vi "Calculate Time and Date.vi"() -> (1 "Date":dbl, 3 "Time":dbl)   [LabVIEW 2018]
doc: "OSDS Calculate Time and Date.vi\n\n This VI calculates the time and date as double based on the time stamp.\n\nOCC Streaming Data System Version 1.0\nJune, 2007 Original Code Consulting David Thomson\n www.originalcode.com"
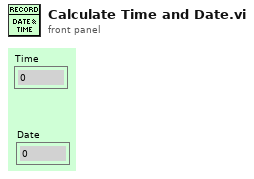
[diagram p1: front panel]
types:
  T1 = typedef "LVDateTimeRec.ctl" = cluster{"fractional second":dbl, "second":i32, "minute":i32, "hour":i32, "day of month":i32, "month":i32, "year":i32, "day of week":i32, "day of year":i32, "DST":i32}
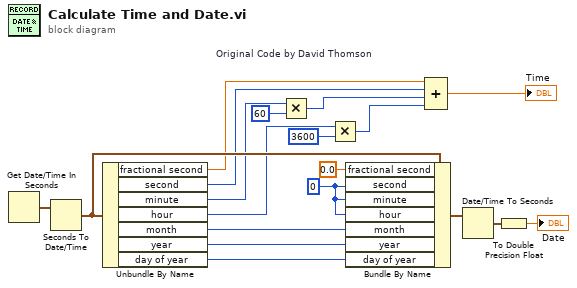
[diagram p0: block diagram]
diagram:
  w16 = 0 ("second")
  n1 = Get Date/Time In Seconds() -> (seconds since 1Jan1904=w19:timestamp)
  n2 = Seconds To Date/Time(time stamp (now)=w19) -> (date time rec=w18:T1)  [unwired: 1 out]
  n3 = Unbundle By Name(w18) -> ("fractional second"=w9:dbl, "second"=w8:i32, "minute"=w7:i32, "hour"=w3:i32, "month"=w14:i32, "year"=w13:i32, "day of year"=w15:i32)
  n4 = Multiply(x=w7, y=60) -> (x*y=w5:i32)
  n5 = Multiply(x=w3, y=3600) -> (x*y=w2:i32)
  n6 = Bundle By Name(cluster=w18, "fractional second"=0.0, "second"=w16, "minute"=w16, "hour"=w16, "month"=w14, "year"=w13, "day of year"=w15) -> (w12:T1)
  n7 = Compound Arithmetic op=ADD "Original Code by David Thomson"(w9, w8, w5, w2) -> (→"Time":dbl)
  n8 = Date/Time To Seconds(2:w12) -> (0:w11:timestamp)  [unwired: 1 out]
  n9 = To Double Precision Float(number=w11) -> (double precision float=→"Date":dbl)
